vi "CLD 17 GUI number pad.vi"() -> ()   [LabVIEW 2019]
doc: "CLD 17\n\nThis VI uses a polling method to respond to changes in the GUI."
uses:
  CLD 17 Keypad_Typedef.ctl
  state_machine.ctl
panel:
  out "error out":errorcluster
  in  "error in (no error)":errorcluster
  out "String":string="0"
  out "Numeric":dbl
  in  "Keypad Cluster":T1
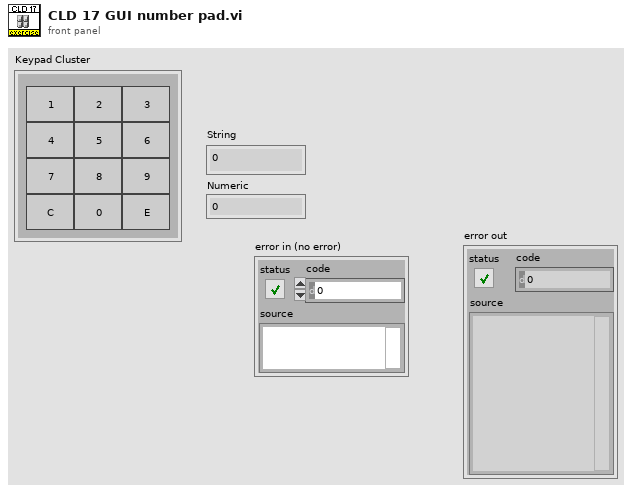
[diagram p1: front panel]
types:
  T1 = typedef "CLD 17 Keypad_Typedef.ctl" = cluster{"0":bool, "1":bool, "2":bool, "3":bool, "4":bool, "5":bool, "6":bool, "7":bool, "8":bool, "9":bool, "C":bool, "E":bool}
  T2 = typedef "state_machine.ctl" = enum16{"initialize", "idle"}
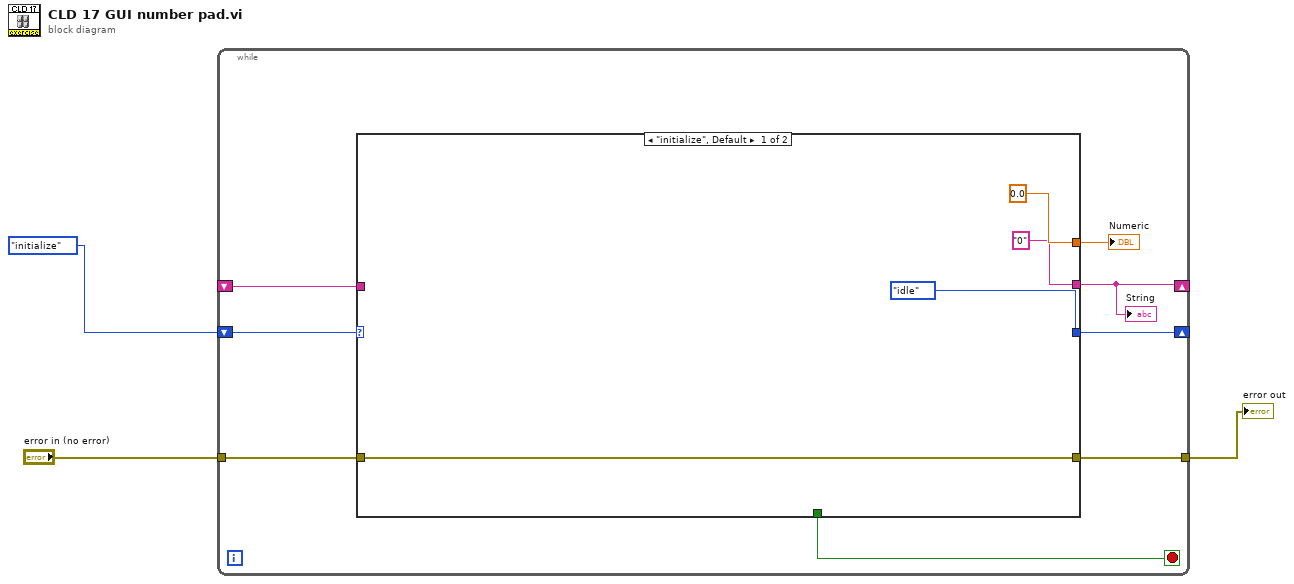
[diagram p0: block diagram]
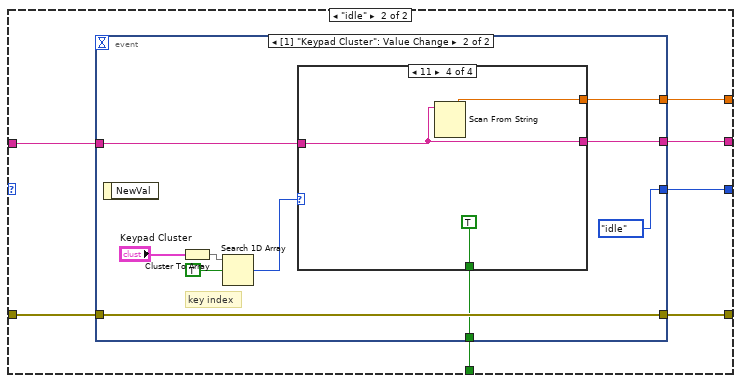
[diagram p2: hidden frame]
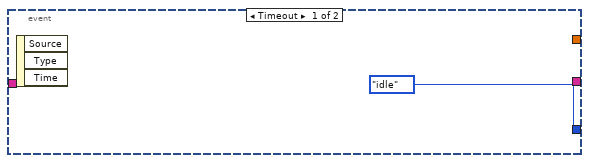
[diagram p3: hidden frame]
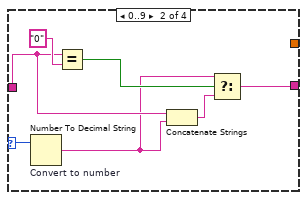
[diagram p5: hidden frame]
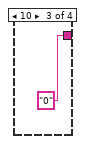
[diagram p6: hidden frame]
diagram:
  n1 = while {
    shift-right: [w10] -> _
    shift-left: state_machine."initialize" -> [w11]
    tunnel: "error in (no error)" -> [w9]
    tunnel: [w8] -> w1
    shift-right: [w5] -> _
    shift-left: _ -> [w4]
    stop <- w7 stop-if-true
    n2 = case shown="\"initialize\", Default" w11 {
      tunnel: [state_machine."idle" w22] -> w10
      tunnel: w9 -> [w15 w21]
      tunnel: [w15 w20] -> w8
      tunnel: [_ w19] -> w7
      tunnel: [0.0 ("Numeric") w16] -> w6
      tunnel: ["0" ("String") w18] -> w5
      tunnel: w4 -> [_ w17]
      frame "initialize", Default {
      }
      frame "idle" {
        n3 = event shown="[1] \"Keypad Cluster\": Value Change" {
          selector: _ -> [_ _]
          dyn-events: _ -> [_ _]
          timeout: _ -> [_ _]
          tunnel: [state_machine."idle" state_machine."idle"] -> w22
          tunnel: w21 -> [_ w33]
          tunnel: [_ w33] -> w20
          tunnel: [_ w26] -> w19
          tunnel: [_ w28] -> w18
          tunnel: w17 -> [_ w27]
          tunnel: [_ w25] -> w16
          event Timeout {
            n4 = event-data() -> ()  [unwired: 1 in, 3 out]
          }
          event Value Change {
            # "key index"
            n5 = event-data() -> ()  [unwired: 1 in, 1 out]
            n6 = Cluster To Array(cluster="Keypad Cluster") -> (array=w32:bool[])
            n7 = Search 1D Array(1D array=w32, element=TRUE) -> (index of element=w29:i32)  [unwired: 1 in]
            n8 = case shown="11" w29 {
              selector: w29 -> [_ w41 _ _]
              tunnel: [w34 w35 "0" w44] -> w28
              tunnel: w27 -> [w34 w38 _ w44]
              tunnel: [_ _ _ TRUE] -> w26
              tunnel: [_ _ _ w43] -> w25
              frame Default {
              }
              frame 0..9 {
                n9 = Number To Decimal String "Convert to number"(number=w41) -> (decimal integer string=w37:string)  [unwired: 1 in]
                n10 = Equal?(x=w38, y="0") -> (x = y?=w39:bool)
                n11 = Concatenate Strings(w38, w37) -> (w36:string)
                n12 = Select(t=w37, s=w39, f=w36) -> (s? t:f=w35:string)
              }
              frame 10 {
              }
              frame 11 {
                n13 = Scan From String(input string=w44) -> (output 1=w43:dbl)  [unwired: 4 in, 3 out]
              }
            }
          }
        }
      }
    }
    "Numeric" <- w6
    "String" <- w5
  }
  "error out" <- w1
